vi "VARIADOR DE FRECUENCIA.vi"() -> ()   [LabVIEW 2017]
uses:
  <vilib>/Instr/_visa.llb/VISA Configure Serial Port (Instr).vi
panel:
  out "x != y?":bool
  out "x .and. y?":bool
  in  "Boolean":bool
  out "Numeric 4":dbl
  out "Numeric 3":dbl
  in  "Puerto":refnum<visa-resource-name>="COM3"
  out "indicador de llegada de datos":bool
  out "String":string
  in  "x":i32
  in  "y":i32
  in  "stop":bool
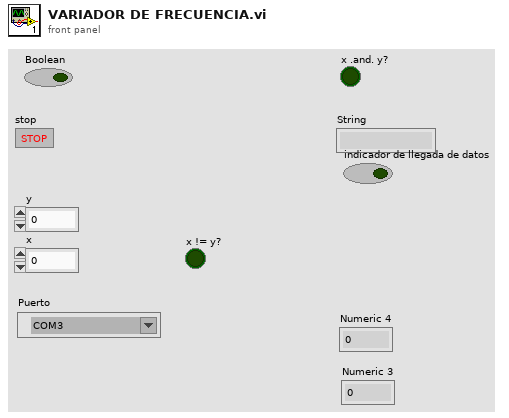
[diagram p1: front panel]
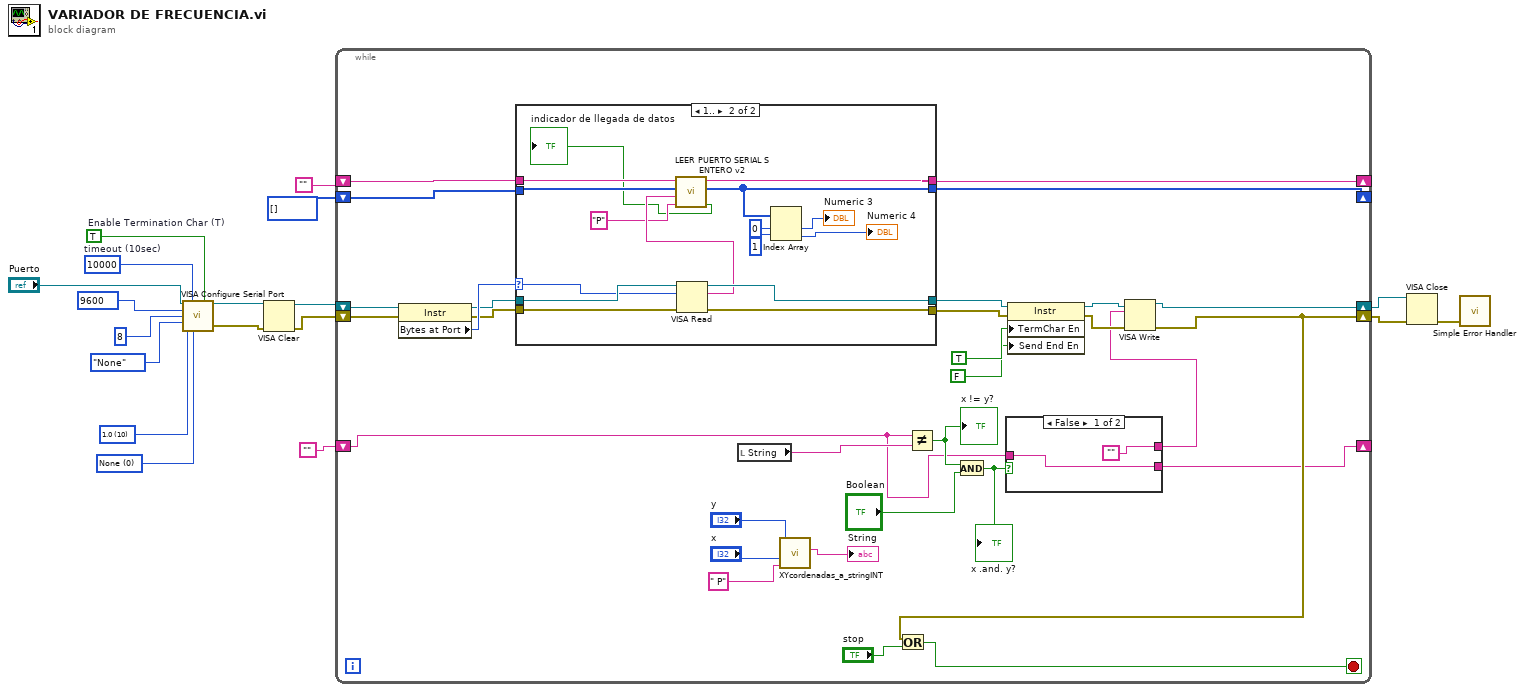
[diagram p0: block diagram]
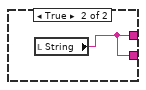
[diagram p2: hidden frame]
diagram:
  w4 = 9600 items=["9600"=9600, "19200"=19200, "38400"=38400, "57600"=57600, "74880"=74880, "115200"=115200] ("BaudRate")
  w7 = u16 10 items=["1.0"=10, "1.5"=15, "2.0"=20] ("stop bits (10: 1 bit)")
  w8 = u16 0 items=["None", "XON/XOFF", "RTS/CTS", "XON/XOFF & RTS/CTS", "DTR/DSR", "XON/XOFF & DTR/DSR"] ("flow control (0:none)")
  w10 = TRUE  # Enable Termination Char (T)
  w11 = u32 10000  # timeout (10sec)
  n1 = call-poly "VISA Configure Serial Port"("VISA resource name"="Puerto", "timeout (10sec)"=w11, "Enable Termination\nChar (T)"=w10, "baud rate (9600)"=w4, "data bits (8)"=u16 8 ("Data bits (8)"), "parity (0:none)"=enum16{"None", "Odd", "Even", "Mark", "Space"}."None" ("Parity (0:none)"), "stop bits (10: 1 bit)"=w7, "flow control (0:none)"=w8) -> ("VISA resource name out"=w3:refnum<visa-resource-name>, "error out"=w2:errorcluster)  [unwired: 6 in]
  n2 = VISA Clear(VISA resource name=w3, error in (no error)=w2) -> (VISA resource name out=w16:refnum<visa-resource-name>, error out=w15:errorcluster)
  n3 = while {
    shift-right: [w41] -> _
    shift-left: "" -> [w48]
    shift-right: [w40] -> _
    shift-left: i32[] [] -> [w42]
    shift-right: [w37] -> w12
    shift-left: w16 -> [w44]
    shift-right: [w36] -> w13
    shift-left: w15 -> [w43]
    shift-right: [w21] -> _
    shift-left: "" -> [w20]
    stop <- w39 stop-if-true
    n4 = property class="Instr"(reference=w44, error in=w43) -> (reference out=w46:refnum<visa-resource-name>, error out=w45:errorcluster, "Bytes at Port"=w47:u32)
    n5 = case shown="1.." w47 {
      selector: w47 -> [_ w67]
      tunnel: w48 -> [w55 w61]
      tunnel: w46 -> [w53 w69]
      tunnel: w45 -> [w52 w68]
      tunnel: w42 -> [w54 w60]
      tunnel: [w55 w62] -> w41
      tunnel: [w54 w56] -> w40
      tunnel: [w53 w71] -> w31
      tunnel: [w52 w70] -> w30
      frame 0, Default {
      }
      frame 1.. {
        n6 = VISA Read(VISA resource name=w69, byte count=w67, error in (no error)=w68) -> (VISA resource name out=w71:refnum<visa-resource-name>, read buffer=w59:string, error out=w70:errorcluster)  [unwired: 1 out]
        n7 = call <userlib>:"LEER PUERTO SERIAL S ENTERO v2.vi"("caracter terminador"="P", "read buffer"=w59, "buffer de datos"=w60, "buffer in"=w61) -> ("indicador de llegada de datos"=→"indicador de llegada de datos":bool, "salida datos numericos"=w56:i32[], "buffer out"=w62:string)  [unwired: 1 in]
        n8 = Index Array(array=w56, index #1=0 ("index"), index #2=1 ("index")) -> (element #1=→"Numeric 3":i32, element #2=→"Numeric 4":i32)
      }
    }
    n9 = local read "String"() -> (w26:string)
    n10 = call "XYcordenadas_a_stringINT.vi"("fin de cadena"=" P", "y"="y", "x"="x") -> ("String"=→"String":string)  [unwired: 7 in, 1 out]
    n11 = Not Equal?(x=w20, y=w26) -> (x != y?=w28:bool)
    "x != y?" <- w28
    n12 = And(x=w28, y="Boolean") -> (x .and. y?=w29:bool)
    "x .and. y?" <- w29
    n13 = case shown="False" w29 {
      tunnel: ["" w51] -> w19
      tunnel: [w49 w51] -> w21
      tunnel: w20 -> [w49 _]
      frame False {
      }
      frame True {
        n14 = local read "String"() -> (w51:string)
      }
    }
    n15 = property class="Instr"(reference=w31, error in=w30, "TermChar En"=TRUE ("Message Based Settings:Termination Character Enable"), "Send End En"=FALSE ("Message Based Settings:Send End Enable")) -> (reference out=w33:refnum<visa-resource-name>, error out=w32:errorcluster)
    n16 = VISA Write(VISA resource name=w33, write buffer=w19, error in (no error)=w32) -> (VISA resource name out=w37:refnum<visa-resource-name>, error out=w36:errorcluster)  [unwired: 1 out]
    n17 = Or(x=w36, y="stop") -> (x .or. y?=w39:bool)
  }
  n18 = VISA Close(VISA resource name=w12, error in (no error)=w13) -> (error out=w14:errorcluster)
  n19 = call <vilib>:"Simple Error Handler.vi"("error in (no error)"=w14) -> ()  [unwired: 4 in, 5 out]
